vi "VTx_control_K2.vi"(4 "VTx_Voltage":dbl, 6 "VTxIndex_In":i8, 7 "SystemPulerSelA":i16, 8 "error in (no error)":errorcluster, 9 "CW/SCW":bool, 10 "Timeout (ms)":i32=40000000, 11 "connection ID in":refnum<k5>) -> (0 "error out":errorcluster, 3 "connection ID out":refnum<k5>)   [LabVIEW 2016]
uses:
  TemperatureMeasure/Thermal_type.vi
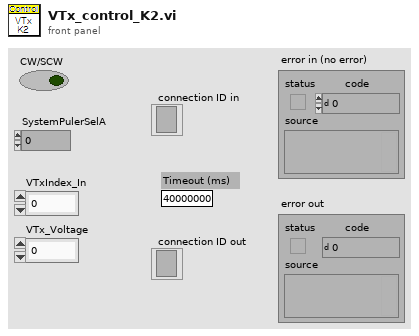
[diagram p1: front panel]
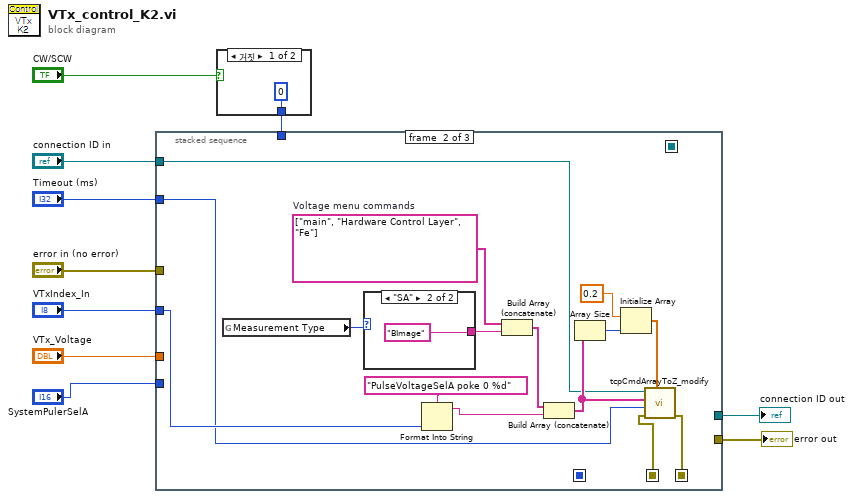
[diagram p0: block diagram]
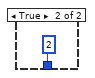
[diagram p2: hidden frame]
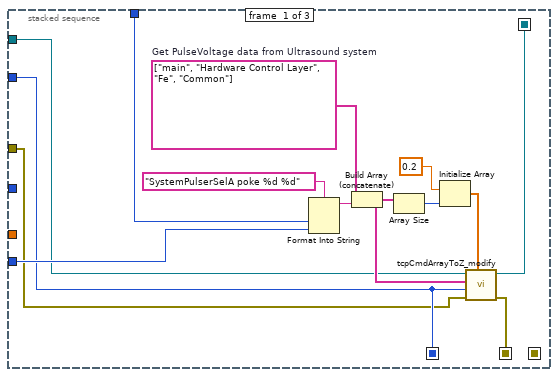
[diagram p3: hidden frame]
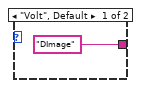
[diagram p4: hidden frame]
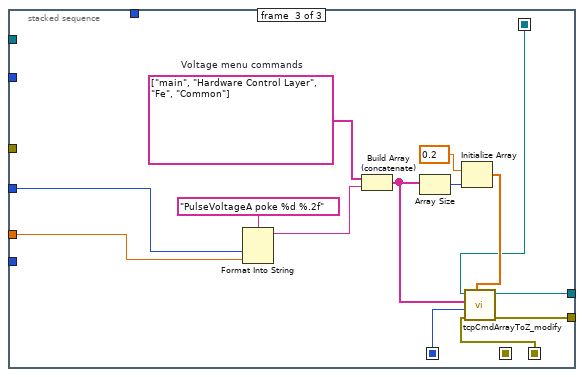
[diagram p5: hidden frame]
diagram:
  n1 = case shown="거짓" "CW/SCW" {
    tunnel: [0 2] -> w8
    frame False {
    }
    frame True {
    }
  }
  n2 = stacked-sequence {
    seq-local: [w14 _ _] -> [_ _ w50]
    seq-local: [w23 _ _] -> [_ w28 _]
    seq-local: [w22 _ _] -> [_ _ w47]
    seq-local: [_ w27 _] -> [_ _ w44]
    tunnel: "VTxIndex_In" -> [_ w31 w49]
    tunnel: "VTx_Voltage" -> [_ _ w48]
    tunnel: w8 -> [w17 _ _]
    tunnel: "SystemPulerSelA" -> [w16 _ _]
    tunnel: "connection ID in" -> [w15 w30 _]
    tunnel: "Timeout (ms)" -> [w14 w29 _]
    tunnel: "error in (no error)" -> [w13 _ _]
    tunnel: [_ _ w46] -> w2
    tunnel: [_ _ w45] -> w1
    frame #0 {
      w20 = string[] ["main", "Hardware Control Layer", "Fe", "Common"]  # Get PulseVoltage data from Ultrasound system
      n3 = Format Into String(format string="SystemPulserSelA poke %d %d" ("Format String"), w17, w16) -> (resulting string=w21:string)  [unwired: 2 in, 1 out]
      n4 = Build Array (concatenate)(w20, w21) -> (w18:string[])
      n5 = Array Size(array=w18) -> (size(s)=w26:i32)
      n6 = Initialize Array(0.2 ("원소"), w26) -> (w24:dbl[])
      n7 = call "tcpCmdArrayToZ_modify.vi"("Delay (sec)"=w24, "error in (no error)"=w13, "Timeout (ms)"=w14, "Command array"=w18, "connection ID in"=w15) -> ("error out"=w23:errorcluster, "connection ID out"=w22:refnum<k5>)  [unwired: 2 in, 3 out]
    }
    frame #1 {
      w32 = string[] ["main", "Hardware Control Layer", "Fe"]  # Voltage menu commands
      n8 = global read "Thermal_type.vi" "Measurement Type"() -> (w41:enum32{"Volt", "SA"})
      n9 = case shown="\"SA\"" w41 {
        tunnel: ["DImage" "BImage"] -> w40
        frame "Volt", Default {
        }
        frame "SA" {
        }
      }
      n10 = Format Into String(format string="PulseVoltageSelA poke 0 %d" ("포맷 문자열"), w31) -> (resulting string=w38:string)  [unwired: 2 in, 1 out]
      n11 = Build Array (concatenate)(w32, w40) -> (w37:string[])
      n12 = Build Array (concatenate)(w37, w38) -> (w33:string[])
      n13 = Array Size(array=w33) -> (size(s)=w36:i32)
      n14 = Initialize Array(0.2 ("원소"), w36) -> (w34:dbl[])
      n15 = call "tcpCmdArrayToZ_modify.vi"("Delay (sec)"=w34, "error in (no error)"=w28, "Timeout (ms)"=w29, "Command array"=w33, "connection ID in"=w30) -> ("error out"=w27:errorcluster)  [unwired: 2 in, 4 out]
    }
    frame #2 {
      w52 = string[] ["main", "Hardware Control Layer", "Fe", "Common"]  # Voltage menu commands
      n16 = Format Into String(format string="PulseVoltageA poke %d %.2f" ("Format String"), w49, w48) -> (resulting string=w53:string)  [unwired: 2 in, 1 out]
      n17 = Build Array (concatenate)(w52, w53) -> (w57:string[])
      n18 = Array Size(array=w57) -> (size(s)=w54:i32)
      n19 = Initialize Array(0.2 ("element"), w54) -> (w56:dbl[])
      n20 = call "tcpCmdArrayToZ_modify.vi"("Delay (sec)"=w56, "error in (no error)"=w44, "Timeout (ms)"=w50, "Command array"=w57, "connection ID in"=w47) -> ("error out"=w45:errorcluster, "connection ID out"=w46:refnum<k5>)  [unwired: 2 in, 3 out]
    }
  }
  "connection ID out" <- w2
  "error out" <- w1
